vi "Wenhch Main.vi"(4 "stop wenching back":bool, 6 "Catapult Clear":bool, 8 "catapult to shift in":T14, 9 "arm button":bool, 10 "Trigger":bool, 11 "Catapult devrevs":T1) -> (0 "catapult to shift out":T14, 1 "Ready To Fire":bool)   [LabVIEW 2013]
uses:
  catapult shift.ctl
  cataplut states.ctl
  catapult type def.ctl
  <vilib>/Rock Robotics/WPI/MotorControl/WPI_MotorControlDeviceRef.ctl
  <vilib>/Rock Robotics/SystemInterfaces/Typedef/FPGA_TypedefDigitalModule.ctl
  <vilib>/Rock Robotics/SystemInterfaces/DIO/FPGA_DIOPWMChannel.ctl
  <vilib>/Rock Robotics/WPI/PWM/WPI_PWMDeadband.ctl
  <vilib>/Rock Robotics/WPI/CAN/Jaguar/SubVIs/WPI_CANJaguar_ControlMode.ctl
  <vilib>/Rock Robotics/WPI/PWM/WPI_PWMTransform_ConPane.ctl
  <vilib>/Rock Robotics/WPI/Solenoid/WPI_SolenoidDevRef.ctl
  <vilib>/Rock Robotics/SystemInterfaces/Typedef/FPGA_TypedefSolenoidModule.ctl
  <vilib>/Rock Robotics/WPI/Solenoid/WPI_SolenoidChannel.ctl
  <vilib>/Rock Robotics/WPI/DigitalInput/WPI_DigitalInputDevRef.ctl
  <vilib>/Rock Robotics/SystemInterfaces/DIO/FPGA_DIOChannel.ctl
  <vilib>/Rock Robotics/WPI/Solenoid/WPI_SolenoidValue.ctl
  <vilib>/Rock Robotics/WPI/Solenoid/WPI_SolenoidSetEnum.vi
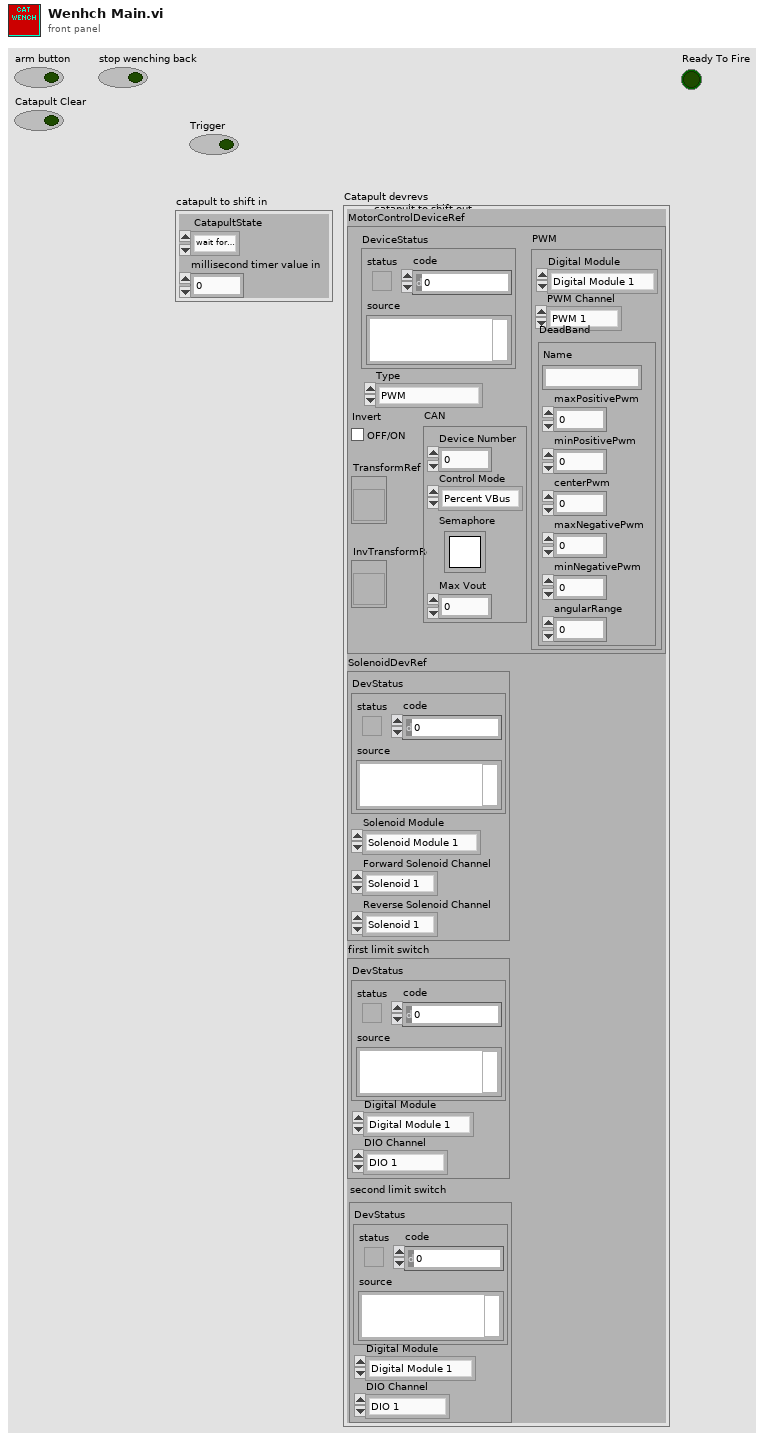
[diagram p1: front panel]
types:
  T1 = typedef "catapult type def.ctl" = cluster{"MotorControlDeviceRef":T2, "SolenoidDevRef":T9, "first limit switch":T12, "second limit switch":T12}
  T2 = typedef "WPI_MotorControlDeviceRef.ctl" = cluster{"DeviceStatus":errorcluster, "Type":enum16{"PWM", "CAN"}, "PWM":cluster{"Digital Module":T3, "PWM Channel":T4, "DeadBand":T5}, "CAN":cluster{"Device Number":u8, "Control Mode":T6, "Semaphore":T7, "Max Vout":dbl}, "Invert":bool, "TransformRef":T8, "InvTransformRef":T8}
  T3 = typedef "FPGA_TypedefDigitalModule.ctl" = enum16{"Digital Module 1", "Digital Module 2"}
  T4 = typedef "FPGA_DIOPWMChannel.ctl" = enum8{"PWM 1", "PWM 2", "PWM 3", "PWM 4", "PWM 5", "PWM 6", "PWM 7", "PWM 8", "PWM 9", "PWM 10", "Invalid"}
  T5 = typedef "WPI_PWMDeadband.ctl" = cluster{"Name":string, "maxPositivePwm":i32, "minPositivePwm":i32, "centerPwm":i32, "maxNegativePwm":i32, "minNegativePwm":i32, "angularRange":u16}
  T6 = typedef "WPI_CANJaguar_ControlMode.ctl" = enum8{"Percent VBus", "Current", "Speed", "Position", "Voltage"}
  T7 = typedef "Semaphore RefNum" = refnum<k1>
  T8 = typedef "WPI_PWMTransform_ConPane.ctl" = refnum<vi>
  T9 = typedef "WPI_SolenoidDevRef.ctl" = cluster{"DevStatus":errorcluster, "Solenoid Module":T10, "Forward Solenoid Channel":T11, "Reverse Solenoid Channel":T11}
  T10 = typedef "FPGA_TypedefSolenoidModule.ctl" = enum16{"Solenoid Module 1", "Solenoid Module 2"}
  T11 = typedef "WPI_SolenoidChannel.ctl" = enum8{"Solenoid 1", "Solenoid 2", "Solenoid 3", "Solenoid 4", "Solenoid 5", "Solenoid 6", "Solenoid 7", "Solenoid 8", "Invalid"}
  T12 = typedef "WPI_DigitalInputDevRef.ctl" = cluster{"DevStatus":errorcluster, "DIO Channel":T13, "Digital Module":T3}
  T13 = typedef "FPGA_DIOChannel.ctl" = enum8{"DIO 1", "DIO 2", "DIO 3", "DIO 4", "DIO 5", "DIO 6", "DIO 7", "DIO 8", "DIO 9", "DIO 10", "DIO 11", "DIO 12", "DIO 13", "DIO 14", "Invalid"}
  T14 = typedef "catapult shift.ctl" = cluster{" CatapultState":T15, "millisecond timer value in":u32}
  T15 = typedef "cataplut states.ctl" = enum16{"wait for trigger", "firing", "wait for coming back", "wench back"}
  T16 = typedef "WPI_SolenoidValue.ctl" = enum16{"Off", "On", "Forward", "Reverse"}
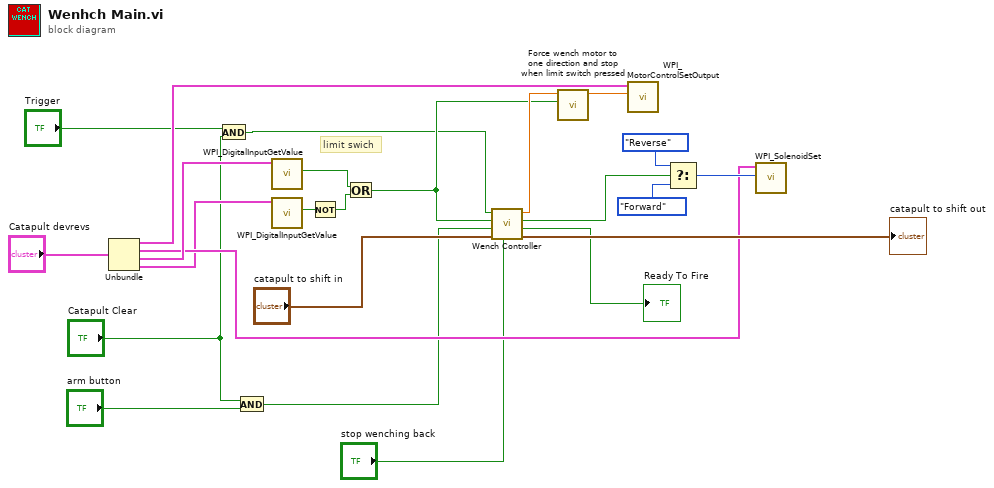
[diagram p0: block diagram]
diagram:
  # "limit swich"
  n1 = Unbundle("Catapult devrevs") -> ("MotorControlDeviceRef"=w15:T2, "SolenoidDevRef"=w16:T9, "first limit switch"=w17:T12, "second limit switch"=w12:T12)
  n2 = And(x="Trigger", y="Catapult Clear") -> (x .and. y?=w5:bool)
  n3 = And(x="Catapult Clear", y="arm button") -> (x .and. y?=w7:bool)
  n4 = call <vilib>:"WPI_DigitalInputGetValue.vi"("DigitalInputDevRef"=w17) -> ("Value"=w3:bool)  [unwired: 8 in, 2 out]
  n5 = call <vilib>:"WPI_DigitalInputGetValue.vi"("DigitalInputDevRef"=w12) -> ("Value"=w11:bool)  [unwired: 8 in, 2 out]
  n6 = Not(x=w11) -> (.not. x?=w2:bool)
  n7 = Or(x=w3, y=w2) -> (x .or. y?=w10:bool)
  n8 = call "Wench Controller.vi"("stop wenching back"="stop wenching back", "catapult from shift"="catapult to shift in", "arm button"=w7, "LimitSwich"=w10, "Trigger"=w5) -> ("catapult to shift"=→"catapult to shift out":T14, "Ready To Fire"=→"Ready To Fire":bool, "Cylinder output"=w21:bool, "Motor output"=w14:dbl)  [unwired: 3 in]
  n9 = call "Force wench motor to one direction and stop when limit switch pressed.vi"("Limit switch input"=w10, "Wench motor input"=w14) -> ("Wench Motor outut"=w13:dbl)  [unwired: 9 in]
  n10 = call <vilib>:"WPI_MotorControlSetOutput.vi"("Output"=w13, "MotorControlDevRef"=w15) -> ()  [unwired: 7 in, 3 out]
  n11 = Select(t=WPI_SolenoidValue."Reverse" ("Value"), s=w21, f=WPI_SolenoidValue."Forward" ("Value")) -> (s? t:f=w24:T16)
  n12 = call-poly <vilib>:"WPI_SolenoidSet.vi"("Value"=w24, "SolenoidDevRef"=w16) -> ()  [unwired: 8 in, 2 out]
